vi "RadioFM.vi"() -> ()   [LabVIEW 2019]
uses:
  <vilib>/Analysis/3filter.llb/Filter Passband Type.ctl
  <vilib>/Waveform/WDTOps.llb/WDT Get Waveform Time Array DBL.vi
  <vilib>/Analysis/3filter.llb/Butterworth Filter (DBL).vi
  <vilib>/measure/maspectr.llb/FFT Power Spectrum and PSD for 1 Chan.vi
  <vilib>/Waveform/WDTOps.llb/WDT Waveform Duration DBL.vi
  <vilib>/Waveform/WDTOps.llb/WDT Get Waveform Subset DBL.vi
  <vilib>/measure/NI_MABase.lvlib
  <vilib>/measure/NI_MAPro.lvlib
  <vilib>/Analysis/NI_AALBase.lvlib
  <vilib>/Analysis/NI_AALPro.lvlib
panel:
  out "Sampling Info":cluster{dbl, dbl}={705600.0, 1411200.0}
  out "dt":dbl=1.417233560090703e-06
  in  "Tab Control 2":T1(tab)
  out "Espectro del Canal":cluster{"f0":dbl, "df":dbl, "magnitude":dbl[]}(graph)={"f0"=0.0, "df"=0.5, "magnitude"=[]}
  out "Espectro Recibido":cluster{"f0":dbl, "df":dbl, "magnitude":dbl[]}(graph)={"f0"=0.0, "df"=0.5, "magnitude"=[]}
  out "Señal Recibida":waveform(dbl)(graph)={"t0"=timestamp(0 s since 1904-01-01), "dt"=1.417233560090703e-06, "Y"=[]}
  out "Espectro Mezclador":cluster{"f0":dbl, "df":dbl, "magnitude":dbl[]}(graph)={"f0"=0.0, "df"=0.5, "magnitude"=[]}
  out "Espectro Detectado":cluster{"f0":dbl, "df":dbl, "magnitude":dbl[]}(graph)={"f0"=0.0, "df"=0.5, "magnitude"=[]}
  out "Señal Detectada":waveform(dbl)(graph)={"t0"=timestamp(0 s since 1904-01-01), "dt"=1.417233560090703e-06, "Y"=[]}
  out "Señal Recuperada":waveform(dbl)(graph)={"t0"=timestamp(0.4 s since 1904-01-01), "dt"=1.417233560090703e-06, "Y"=[]}
  out "Espectro Recuperado":cluster{"f0":dbl, "df":dbl, "magnitude":dbl[]}(graph)={"f0"=0.0, "df"=0.6250005536073497, "magnitude"=[]}
  in  "Sintonizador":cluster{"Emisora":dbl, "Volumen":dbl}={"Emisora"=65050.0, "Volumen"=5.081596097153018} {"Volumen" scale=0.0..10.0; "Emisora" scale=44050.0..65050.0}
  in  "stop":bool
  in  "Tab Control":enum32{"Page 1", "Page 2", "Page 3", "Page 4"}(tab)
  out "Beta":dbl=0.003302742812078559
  out "Espectro Emisora":cluster{"f0":dbl, "df":dbl, "magnitude":dbl[]}(graph)={"f0"=0.0, "df"=0.5, "magnitude"=[]}
  in  "Mensaje 1":T2={"Fase"=0.0, "Frecuencia"=1513.8932349543995, "Amplitud"=5.617529880478088, "Kf"=5.0} {"Amplitud" scale=0.0..100.0; "Frecuencia" scale=1.0..5000.0; "Fase" scale=0.0..90.0}
  out "Emisora 1":waveform(dbl)(graph)={"t0"=timestamp(232 s since 1904-01-01), "dt"=1.417233560090703e-06, "Y"=[]}
  out "Beta 2":dbl=16.18677363495819
  out "Emisora 2":waveform(dbl)(graph)={"t0"=timestamp(232 s since 1904-01-01), "dt"=1.417233560090703e-06, "Y"=[]}
  in  "Mensaje 2":T2={"Fase"=0.0, "Frecuencia"=308.8941695707426, "Amplitud"=5.0199203187251, "Kf"=5000.0} {"Amplitud" scale=0.0..100.0; "Frecuencia" scale=0.0..1000.0; "Fase" scale=0.0..10.0}
  out "Espectro Emisora 2":cluster{"f0":dbl, "df":dbl, "magnitude":dbl[]}(graph)={"f0"=0.0, "df"=0.5, "magnitude"=[]}
  out "Beta 3":dbl=14.81360563253253
  out "Emisora 3":waveform(dbl)(graph)={"t0"=timestamp(232 s since 1904-01-01), "dt"=1.417233560090703e-06, "Y"=[]}
  in  "Mensaje 3":T2={"Fase"=0.0, "Frecuencia"=337.5275489324068, "Amplitud"=5.0199203187251, "Kf"=5000.0} {"Amplitud" scale=0.0..100.0; "Frecuencia" scale=0.0..1000.0; "Fase" scale=0.0..10.0}
  out "Espectro Emisora 3":cluster{"f0":dbl, "df":dbl, "magnitude":dbl[]}(graph)={"f0"=0.0, "df"=0.5, "magnitude"=[]}
  out "Beta 4":dbl=0.058823529411764705
  out "Emisora 4":waveform(dbl)(graph)={"t0"=timestamp(0 s since 1904-01-01), "dt"=1.417233560090703e-06, "Y"=[]}
  in  "Mensaje 4":cluster{"Amplitud":dbl, "Kf":dbl}={"Amplitud"=5.016722408026756, "Kf"=200.0} {"Amplitud" scale=0.0..100.0}
  out "Espectro Emisora 4":cluster{"f0":dbl, "df":dbl, "magnitude":dbl[]}(graph)={"f0"=0.0, "df"=0.4778519417475728, "magnitude"=[]}
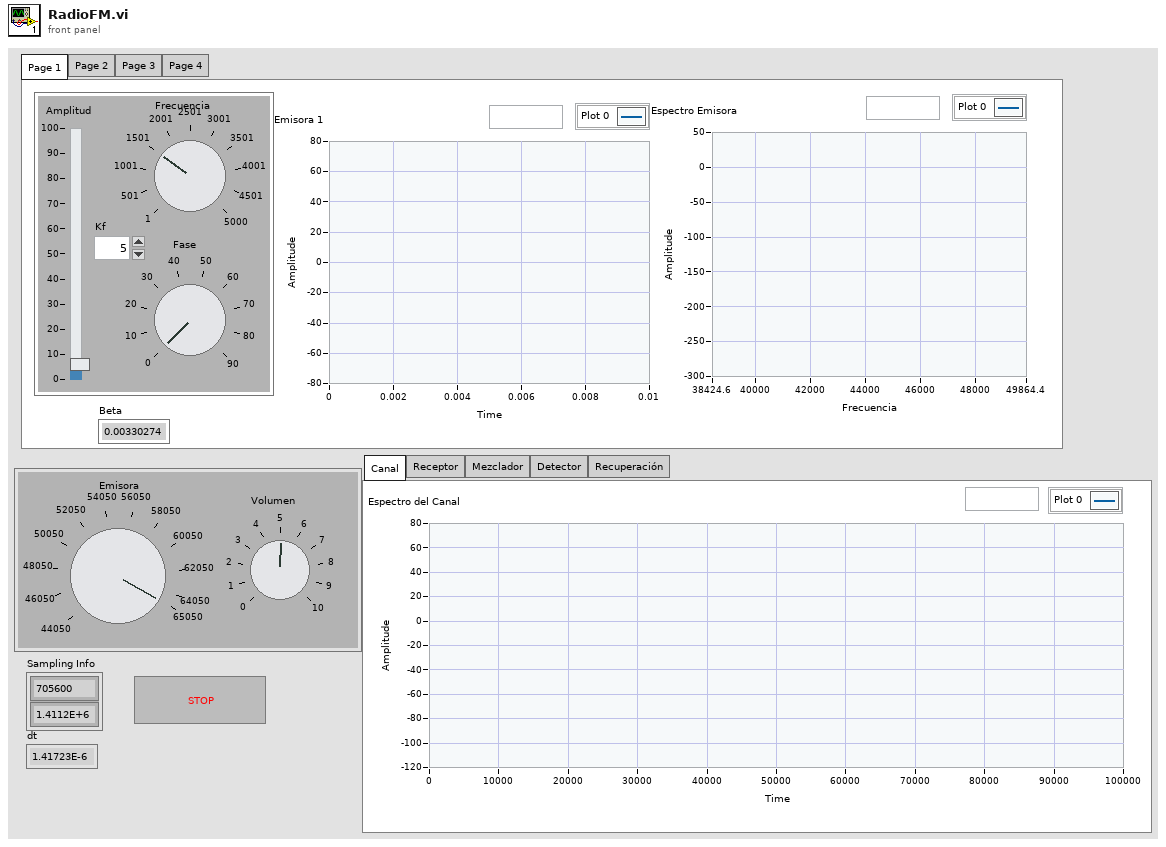
[diagram p1: front panel]
types:
  T1 = enum32{"Canal", "Receptor", "Mezclador", "Detector", "Recuperación"}
  T2 = cluster{"Fase":dbl, "Frecuencia":dbl, "Amplitud":dbl, "Kf":dbl}
  T3 = typedef "NI_AALBase.lvlib/Filter Passband Type.ctl" = enum32{"Lowpass", "Highpass", "Bandpass", "Bandstop"}
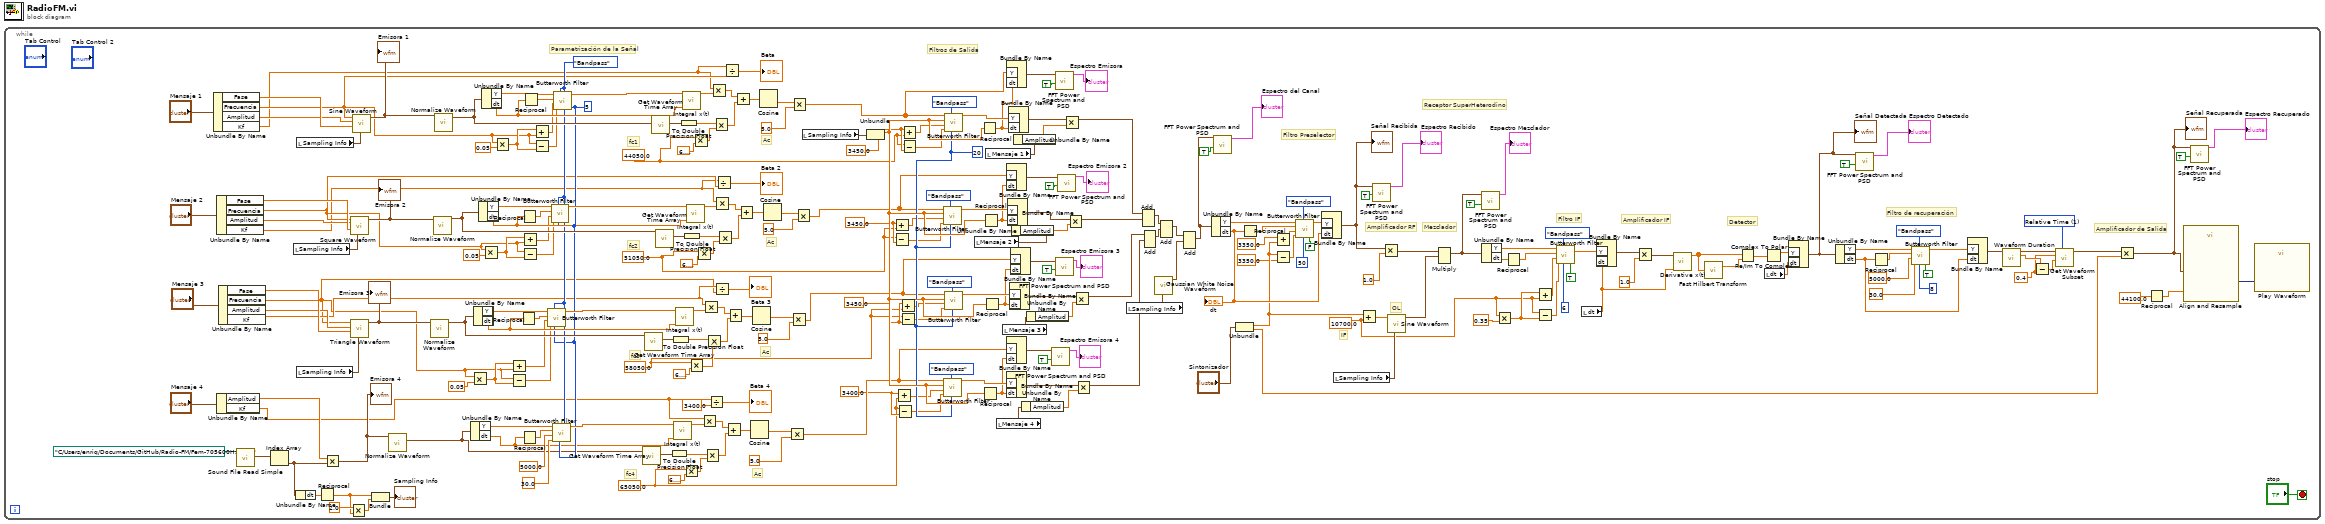
[diagram p0: block diagram]
diagram:
  n1 = while {
    stop <- "stop" stop-if-true
    w15 = 44050.0 ("y")
    w20 = 3450.0 ("x")
    w16 = 51050.0 ("x")
    w23 = 3450.0 ("x+y")
    w17 = 58050.0 ("y")
    w27 = 3450.0 ("y")
    w26 = 3400.0 ("y")
    w18 = 65050.0
    w43 = u16 1 items=["Samples", "Relative Time"] ("start/duration format")
    w49 = 0.4 ("start samples/time")
    w102 = 5 ("order")
    w107 = Filter_Passband_Type."Bandpass" ("filter type")
    w160 = 20 ("order")
    w80 = 10700.0 ("y")
    # "Amplificador de Salida"
    # "Parametrización de la Señal"
    # "Filtro IF"
    # "Filtro de recuperación"
    # "Amplificador RF"
    # "Amplificador IF"
    # "Detector"
    # "Mezclador"
    # "Receptor SuperHeterodino"
    # "Filtros de Salida"
    # "Ac"
    # "fc4"
    # "Ac"
    # "fc3"
    # "Ac"
    # "fc2"
    # "Ac"
    # "fc1"
    # "Filtro Preselector"
    # "IF"
    # "OL"
    n2 = Unbundle By Name("Mensaje 1") -> ("Fase"=w218:dbl, "Frecuencia"=w63:dbl, "Amplitud"=w210:dbl, "Kf"=w62:dbl)
    n3 = Unbundle By Name("Mensaje 2") -> ("Fase"=w216:dbl, "Frecuencia"=w61:dbl, "Amplitud"=w197:dbl, "Kf"=w60:dbl)
    n4 = Unbundle By Name("Mensaje 4") -> ("Amplitud"=w211:dbl, "Kf"=w57:dbl)
    n5 = Unbundle By Name("Mensaje 3") -> ("Fase"=w214:dbl, "Frecuencia"=w58:dbl, "Amplitud"=w171:dbl, "Kf"=w59:dbl)
    n6 = call <vilib>:"Sound File Read Simple.vi"("path"=path "C:/Users/enriq/Documents/GitHub/Radio-FM/Fem-705600Hz.wav") -> ("data"=w257:waveform(dbl)[])  [unwired: 7 in, 3 out]
    n7 = Index Array(array=w257) -> (element=w212:waveform(dbl))  [unwired: 1 in]
    n8 = local read "Sampling Info"() -> (w241:cluster{dbl, dbl})
    n9 = Unbundle By Name(w212) -> ("dt"=w256:dbl)
    n10 = local read "Sampling Info"() -> (w242:cluster{dbl, dbl})
    n11 = local read "Sampling Info"() -> (w253:cluster{dbl, dbl})
    n12 = Reciprocal(x=w256) -> (1/x=w170:dbl)
    n13 = Multiply(x=w211, y=w212) -> (x*y=w72:waveform(dbl))
    "Emisora 4" <- w72
    n14 = Multiply(x=2.0, y=w170) -> (x*y=w254:dbl)
    n15 = call <vilib>:"Square Waveform.vi"("sampling info"=w241, "phase"=w216, "amplitude"=w197, "frequency"=w61) -> ("signal out"=w196:waveform(dbl))  [unwired: 6 in, 1 out]
    "Emisora 2" <- w196
    n16 = call <vilib>:"Triangle Waveform.vi"("sampling info"=w242, "phase"=w214, "amplitude"=w171, "frequency"=w58) -> ("signal out"=w172:waveform(dbl))  [unwired: 6 in, 1 out]
    "Emisora 3" <- w172
    n17 = call <vilib>:"Sine Waveform.vi"("sampling info"=w253, "phase"=w218, "amplitude"=w210, "frequency"=w63) -> ("signal out"=w139:waveform(dbl))  [unwired: 6 in, 1 out]
    "Emisora 1" <- w139
    n18 = Bundle(w170, w254) -> (→"Sampling Info":cluster{dbl, dbl})  [unwired: 1 in]
    n19 = call <vilib>:"Normalize Waveform.vi"("waveform in"=w72) -> ("normalized waveform"=w44:waveform(dbl))  [unwired: 7 in, 3 out]
    n20 = call <vilib>:"Normalize Waveform.vi"("waveform in"=w172) -> ("normalized waveform"=w136:waveform(dbl))  [unwired: 7 in, 3 out]
    n21 = call <vilib>:"Normalize Waveform.vi"("waveform in"=w196) -> ("normalized waveform"=w137:waveform(dbl))  [unwired: 7 in, 3 out]
    n22 = call <vilib>:"Normalize Waveform.vi"("waveform in"=w139) -> ("normalized waveform"=w138:waveform(dbl))  [unwired: 7 in, 3 out]
    n23 = Unbundle By Name(w44) -> ("Y"=w173:dbl[], "dt"=w78:dbl)
    n24 = Multiply(x=w58, y=0.05) -> (x*y=w123:dbl)
    n25 = Unbundle By Name(w136) -> ("Y"=w194:dbl[], "dt"=w115:dbl)
    n26 = Unbundle By Name(w137) -> ("Y"=w198:dbl[], "dt"=w114:dbl)
    n27 = Unbundle By Name(w138) -> ("Y"=w226:dbl[], "dt"=w130:dbl)
    n28 = Multiply(x=w61, y=0.05) -> (x*y=w124:dbl)
    n29 = Multiply(x=w63, y=0.05) -> (x*y=w129:dbl)
    n30 = Add(x=w123, y=w58) -> (x+y=w109:dbl)
    n31 = Subtract(x=w58, y=w123) -> (x-y=w108:dbl)
    n32 = Reciprocal(x=w115) -> (1/x=w117:dbl)
    n33 = Reciprocal(x=w114) -> (1/x=w118:dbl)
    n34 = Reciprocal(x=w78) -> (1/x=w116:dbl)
    n35 = Add(x=w124, y=w61) -> (x+y=w113:dbl)
    n36 = Subtract(x=w61, y=w124) -> (x-y=w112:dbl)
    n37 = Reciprocal(x=w130) -> (1/x=w131:dbl)
    n38 = Add(x=w129, y=w63) -> (x+y=w127:dbl)
    n39 = Subtract(x=w63, y=w129) -> (x-y=w126:dbl)
    n40 = call-poly <vilib>:"Butterworth Filter.vi"("order"=w102, "filter type"=w107, "low cutoff freq: fl"=w108, "high cutoff freq: fh"=w109, "sampling freq: fs"=w117, "X"=w194) -> ("Filtered X"=w120:dbl[])  [unwired: 2 in, 1 out]
    n41 = call-poly <vilib>:"Butterworth Filter.vi"("order"=w102, "filter type"=w107, "low cutoff freq: fl"=w112, "high cutoff freq: fh"=w113, "sampling freq: fs"=w118, "X"=w198) -> ("Filtered X"=w121:dbl[])  [unwired: 2 in, 1 out]
    n42 = call-poly <vilib>:"Butterworth Filter.vi"("order"=w102, "filter type"=w107, "low cutoff freq: fl"=30.0, "high cutoff freq: fh"=5000.0, "sampling freq: fs"=w116, "X"=w173) -> ("Filtered X"=w119:dbl[])  [unwired: 2 in, 1 out]
    n43 = call-poly <vilib>:"Butterworth Filter.vi"("order"=w102, "filter type"=w107, "low cutoff freq: fl"=w126, "high cutoff freq: fh"=w127, "sampling freq: fs"=w131, "X"=w226) -> ("Filtered X"=w132:dbl[])  [unwired: 2 in, 1 out]
    n44 = call-poly <vilib>:"Get Waveform Time Array.vi"("waveform in"=w44) -> ("X array"=w178:timestamp[])  [unwired: 9 in, 1 out]
    n45 = call-poly <vilib>:"Get Waveform Time Array.vi"("waveform in"=w136) -> ("X array"=w189:timestamp[])  [unwired: 9 in, 1 out]
    n46 = call-poly <vilib>:"Get Waveform Time Array.vi"("waveform in"=w138) -> ("X array"=w227:timestamp[])  [unwired: 9 in, 1 out]
    n47 = call-poly <vilib>:"Get Waveform Time Array.vi"("waveform in"=w137) -> ("X array"=w203:timestamp[])  [unwired: 9 in, 1 out]
    n48 = To Double Precision Float(number=w178) -> (double precision float=w177:dbl[])
    n49 = To Double Precision Float(number=w189) -> (double precision float=w190:dbl[])
    n50 = call <vilib>:"Integral x(t).vi"("dt"=w78, "X"=w119) -> ("Integral X"=w179:dbl[])  [unwired: 8 in, 1 out]
    n51 = call <vilib>:"Integral x(t).vi"("dt"=w115, "X"=w120) -> ("Integral X"=w188:dbl[])  [unwired: 8 in, 1 out]
    n52 = To Double Precision Float(number=w227) -> (double precision float=w228:dbl[])
    n53 = call <vilib>:"Integral x(t).vi"("dt"=w130, "X"=w132) -> ("Integral X"=w225:dbl[])  [unwired: 8 in, 1 out]
    n54 = Multiply(x=w18, y=6.283185307179586) -> (x*y=w174:dbl)
    n55 = To Double Precision Float(number=w203) -> (double precision float=w202:dbl[])
    n56 = call <vilib>:"Integral x(t).vi"("dt"=w114, "X"=w121) -> ("Integral X"=w204:dbl[])  [unwired: 8 in, 1 out]
    n57 = Multiply(x=w17, y=6.283185307179586) -> (x*y=w193:dbl)
    n58 = Multiply(x=w15, y=6.283185307179586) -> (x*y=w230:dbl)
    n59 = Multiply(x=w16, y=6.283185307179586) -> (x*y=w199:dbl)
    n60 = Multiply(x=w57, y=w179) -> (x*y=w176:dbl[])
    n61 = Multiply(x=w59, y=w188) -> (x*y=w191:dbl[])
    n62 = Multiply(x=w177, y=w174) -> (x*y=w175:dbl[])
    n63 = Multiply(x=w190, y=w193) -> (x*y=w192:dbl[])
    n64 = Divide(x=w57, y=3400.0) -> (x/y=→"Beta 4":dbl)
    n65 = Multiply(x=w62, y=w225) -> (x*y=w64:dbl[])
    n66 = Multiply(x=w228, y=w230) -> (x*y=w229:dbl[])
    n67 = Multiply(x=w60, y=w204) -> (x*y=w201:dbl[])
    n68 = Divide(x=w59, y=w58) -> (x/y=→"Beta 3":dbl)
    n69 = Divide(x=w60, y=w61) -> (x/y=→"Beta 2":dbl)
    n70 = Multiply(x=w202, y=w199) -> (x*y=w200:dbl[])
    n71 = Divide(x=w62, y=w63) -> (x/y=→"Beta":dbl)
    n72 = Add(x=w176, y=w175) -> (x+y=w180:dbl[])
    n73 = Add(x=w191, y=w192) -> (x+y=w187:dbl[])
    n74 = Add(x=w64, y=w229) -> (x+y=w224:dbl[])
    n75 = Add(x=w201, y=w200) -> (x+y=w205:dbl[])
    n76 = Cosine(x=w180) -> (cos(x)=w181:dbl[])
    n77 = Cosine(x=w187) -> (cos(x)=w186:dbl[])
    n78 = Cosine(x=w224) -> (cos(x)=w223:dbl[])
    n79 = Cosine(x=w205) -> (cos(x)=w206:dbl[])
    n80 = Multiply(x=w181, y=5.0) -> (x*y=w87:dbl[])
    n81 = Multiply(x=w186, y=5.0) -> (x*y=w88:dbl[])
    n82 = Multiply(x=w223, y=5.0) -> (x*y=w142:dbl[])
    n83 = Multiply(x=w206, y=5.0) -> (x*y=w92:dbl[])
    n84 = local read "Sampling Info"() -> (w164:cluster{dbl, dbl})
    n85 = Unbundle(w164) -> (w195:dbl)  [unwired: 1 out]
    n86 = Add(x=w23, y=w16) -> (x+y=w25:dbl)
    n87 = Subtract(x=w16, y=w23) -> (x-y=w24:dbl)
    n88 = Add(x=w26, y=w18) -> (x+y=w31:dbl)
    n89 = Subtract(x=w18, y=w26) -> (x-y=w30:dbl)
    n90 = Add(x=w27, y=w17) -> (x+y=w29:dbl)
    n91 = Subtract(x=w17, y=w27) -> (x-y=w28:dbl)
    n92 = Add(x=w20, y=w15) -> (x+y=w22:dbl)
    n93 = Subtract(x=w15, y=w20) -> (x-y=w21:dbl)
    n94 = call-poly <vilib>:"Butterworth Filter.vi"("order"=w160, "filter type"=Filter_Passband_Type."Bandpass", "low cutoff freq: fl"=w24, "high cutoff freq: fh"=w25, "sampling freq: fs"=w195, "X"=w92) -> ("Filtered X"=w168:dbl[])  [unwired: 2 in, 1 out]
    n95 = call-poly <vilib>:"Butterworth Filter.vi"("order"=w160, "filter type"=Filter_Passband_Type."Bandpass", "low cutoff freq: fl"=w30, "high cutoff freq: fh"=w31, "sampling freq: fs"=w195, "X"=w87) -> ("Filtered X"=w166:dbl[])  [unwired: 2 in, 1 out]
    n96 = call-poly <vilib>:"Butterworth Filter.vi"("order"=w160, "filter type"=Filter_Passband_Type."Bandpass", "low cutoff freq: fl"=w21, "high cutoff freq: fh"=w22, "sampling freq: fs"=w195, "X"=w142) -> ("Filtered X"=w169:dbl[])  [unwired: 2 in, 1 out]
    n97 = call-poly <vilib>:"Butterworth Filter.vi"("order"=w160, "filter type"=Filter_Passband_Type."Bandpass", "low cutoff freq: fl"=w28, "high cutoff freq: fh"=w29, "sampling freq: fs"=w195, "X"=w88) -> ("Filtered X"=w167:dbl[])  [unwired: 2 in, 1 out]
    n98 = local read "Mensaje 2"() -> (w4:T2)
    n99 = Reciprocal(x=w195) -> (1/x=w141:dbl)
    n100 = Reciprocal(x=w195) -> (1/x=w86:dbl)
    n101 = Reciprocal(x=w195) -> (1/x=w91:dbl)
    n102 = Reciprocal(x=w195) -> (1/x=w89:dbl)
    n103 = local read "Mensaje 1"() -> (w2:T2)
    n104 = local read "Mensaje 4"() -> (w8:cluster{"Amplitud":dbl, "Kf":dbl})
    n105 = local read "Mensaje 3"() -> (w6:T2)
    n106 = Bundle By Name("Y"=w92, "dt"=w91) -> (w93:waveform(dbl))  [unwired: 1 in]
    n107 = Bundle By Name("Y"=w87, "dt"=w86) -> (w40:waveform(dbl))  [unwired: 1 in]
    n108 = Bundle By Name("Y"=w166, "dt"=w86) -> (w19:waveform(dbl))  [unwired: 1 in]
    n109 = Bundle By Name("Y"=w142, "dt"=w141) -> (w48:waveform(dbl))  [unwired: 1 in]
    n110 = Bundle By Name("Y"=w168, "dt"=w91) -> (w143:waveform(dbl))  [unwired: 1 in]
    n111 = Bundle By Name("Y"=w169, "dt"=w141) -> (w47:waveform(dbl))  [unwired: 1 in]
    n112 = Bundle By Name("Y"=w167, "dt"=w89) -> (w243:waveform(dbl))  [unwired: 1 in]
    n113 = Bundle By Name("Y"=w88, "dt"=w89) -> (w90:waveform(dbl))  [unwired: 1 in]
    n114 = Unbundle By Name(w4) -> ("Amplitud"=w3:dbl)
    n115 = Unbundle By Name(w2) -> ("Amplitud"=w1:dbl)
    n116 = Unbundle By Name(w8) -> ("Amplitud"=w7:dbl)
    n117 = Unbundle By Name(w6) -> ("Amplitud"=w5:dbl)
    n118 = call-poly <vilib>:"FFT Power Spectrum and PSD.vi"("dB On (F)"=TRUE, "time signal"=w40) -> ("Power Spectrum / PSD"=→"Espectro Emisora 4":cluster{"f0":dbl, "df":dbl, "magnitude":dbl[]})  [unwired: 6 in, 3 out]
    n119 = call-poly <vilib>:"FFT Power Spectrum and PSD.vi"("dB On (F)"=TRUE, "time signal"=w48) -> ("Power Spectrum / PSD"=→"Espectro Emisora":cluster{"f0":dbl, "df":dbl, "magnitude":dbl[]})  [unwired: 6 in, 3 out]
    n120 = call-poly <vilib>:"FFT Power Spectrum and PSD.vi"("dB On (F)"=TRUE, "time signal"=w90) -> ("Power Spectrum / PSD"=→"Espectro Emisora 3":cluster{"f0":dbl, "df":dbl, "magnitude":dbl[]})  [unwired: 6 in, 3 out]
    n121 = call-poly <vilib>:"FFT Power Spectrum and PSD.vi"("dB On (F)"=TRUE, "time signal"=w93) -> ("Power Spectrum / PSD"=→"Espectro Emisora 2":cluster{"f0":dbl, "df":dbl, "magnitude":dbl[]})  [unwired: 6 in, 3 out]
    n122 = Multiply(x=w47, y=w1) -> (x*y=w12:waveform(dbl))
    n123 = Multiply(x=w143, y=w3) -> (x*y=w11:waveform(dbl))
    n124 = Multiply(x=w243, y=w5) -> (x*y=w10:waveform(dbl))
    n125 = Multiply(x=w19, y=w7) -> (x*y=w9:waveform(dbl))
    n126 = local read "Sampling Info"() -> (w103:cluster{dbl, dbl})
    n127 = Add(1:w11, 2:w12) -> (0:w245:waveform(dbl))  [unwired: 1 in, 1 out]
    n128 = Add(1:w9, 2:w10) -> (0:w244:waveform(dbl))  [unwired: 1 in, 1 out]
    n129 = call <vilib>:"Gaussian White Noise Waveform.vi"("sampling info"=w103) -> ("signal out"=w104:waveform(dbl))  [unwired: 9 in, 1 out]
    n130 = Add(1:w244, 2:w245) -> (0:w14:waveform(dbl))  [unwired: 1 in, 1 out]
    n131 = Add(1:w104, 2:w14) -> (0:w13:waveform(dbl))  [unwired: 1 in, 1 out]
    n132 = Unbundle By Name(w13) -> ("Y"=w237:dbl[], "dt"=w140:dbl)
    "dt" <- w140
    n133 = call-poly <vilib>:"FFT Power Spectrum and PSD.vi"("dB On (F)"=TRUE, "time signal"=w13) -> ("Power Spectrum / PSD"=→"Espectro del Canal":cluster{"f0":dbl, "df":dbl, "magnitude":dbl[]})  [unwired: 6 in, 3 out]
    n134 = Unbundle("Sintonizador") -> ("Emisora"=w133:dbl, "Volumen"=w105:dbl)
    n135 = Reciprocal(x=w140) -> (1/x=w236:dbl)
    n136 = Add(x=3350.0, y=w133) -> (x+y=w235:dbl)
    n137 = Subtract(x=w133, y=3350.0) -> (x-y=w165:dbl)
    n138 = call-poly <vilib>:"Butterworth Filter.vi"("init/cont (init:F)"=FALSE, "order"=50, "filter type"=Filter_Passband_Type."Bandpass", "low cutoff freq: fl"=w165, "high cutoff freq: fh"=w235, "sampling freq: fs"=w236, "X"=w237) -> ("Filtered X"=w238:dbl[])  [unwired: 1 in, 1 out]
    n139 = Bundle By Name("Y"=w238, "dt"=w140) -> (w70:waveform(dbl))  [unwired: 1 in]
    "Señal Recibida" <- w70
    n140 = local read "Sampling Info"() -> (w159:cluster{dbl, dbl})
    n141 = Add(x=w133, y=w80) -> (x+y=w234:dbl)
    n142 = call-poly <vilib>:"FFT Power Spectrum and PSD.vi"("dB On (F)"=TRUE, "time signal"=w70) -> ("Power Spectrum / PSD"=→"Espectro Recibido":cluster{"f0":dbl, "df":dbl, "magnitude":dbl[]})  [unwired: 6 in, 3 out]
    n143 = Multiply(x=w70, y=1.0) -> (x*y=w233:waveform(dbl))
    n144 = call <vilib>:"Sine Waveform.vi"("sampling info"=w159, "frequency"=w234) -> ("signal out"=w38:waveform(dbl))  [unwired: 8 in, 1 out]
    n145 = Multiply(1:w38, 2:w233) -> (0:w71:waveform(dbl))  [unwired: 1 in, 1 out]
    n146 = call-poly <vilib>:"FFT Power Spectrum and PSD.vi"("dB On (F)"=TRUE, "time signal"=w71) -> ("Power Spectrum / PSD"=→"Espectro Mezclador":cluster{"f0":dbl, "df":dbl, "magnitude":dbl[]})  [unwired: 6 in, 3 out]
    n147 = Unbundle By Name(w71) -> ("Y"=w154:dbl[], "dt"=w155:dbl)
    n148 = Multiply(x=w80, y=0.35) -> (x*y=w134:dbl)
    n149 = Reciprocal(x=w155) -> (1/x=w153:dbl)
    n150 = Add(x=w134, y=w80) -> (x+y=w152:dbl)
    n151 = Subtract(x=w80, y=w134) -> (x-y=w151:dbl)
    n152 = call-poly <vilib>:"Butterworth Filter.vi"("init/cont (init:F)"=TRUE, "order"=6, "filter type"=Filter_Passband_Type."Bandpass", "low cutoff freq: fl"=w151, "high cutoff freq: fh"=w152, "sampling freq: fs"=w153, "X"=w154) -> ("Filtered X"=w146:dbl[])  [unwired: 1 in, 1 out]
    n153 = local read "dt"() -> (w73:dbl)
    n154 = Bundle By Name("Y"=w146, "dt"=w73) -> (w69:waveform(dbl))  [unwired: 1 in]
    n155 = Multiply(x=w69, y=1.0) -> (x*y=w81:waveform(dbl))
    n156 = call <vilib>:"Derivative x(t).vi"("dt"=w73, "X"=w81) -> ("dX/dt"=w74:dbl[])  [unwired: 8 in, 1 out]
    n157 = call <vilib>:"Fast Hilbert Transform.vi"("X"=w74) -> ("Hilbert{X}"=w76:dbl[])  [unwired: 1 out]
    n158 = Re/Im To Complex(1:w76, 2:w74) -> (0:w77:cdb[])
    n159 = local read "dt"() -> (w145:dbl)
    n160 = Complex To Polar(r * e^(i*theta)=w77) -> (r=w75:dbl[])  [unwired: 1 out]
    n161 = Bundle By Name("Y"=w75, "dt"=w145) -> (w65:waveform(dbl))  [unwired: 1 in]
    "Señal Detectada" <- w65
    n162 = Unbundle By Name(w65) -> ("Y"=w147:dbl[], "dt"=w79:dbl)
    n163 = call-poly <vilib>:"FFT Power Spectrum and PSD.vi"("dB On (F)"=TRUE, "time signal"=w65) -> ("Power Spectrum / PSD"=→"Espectro Detectado":cluster{"f0":dbl, "df":dbl, "magnitude":dbl[]})  [unwired: 6 in, 3 out]
    n164 = Reciprocal(x=w79) -> (1/x=w158:dbl)
    n165 = call-poly <vilib>:"Butterworth Filter.vi"("init/cont (init:F)"=TRUE, "order"=8, "filter type"=Filter_Passband_Type."Bandpass", "low cutoff freq: fl"=30.0, "high cutoff freq: fh"=5000.0, "sampling freq: fs"=w158, "X"=w147) -> ("Filtered X"=w144:dbl[])  [unwired: 1 in, 1 out]
    n166 = Bundle By Name("Y"=w144, "dt"=w79) -> (w35:waveform(dbl))  [unwired: 1 in]
    n167 = call-poly <vilib>:"Waveform Duration.vi"("waveform in"=w35) -> ("duration"=w51:dbl, "waveform out"=w39:waveform(dbl))  [unwired: 8 in, 1 out]
    n168 = Subtract(x=w51, y=w49) -> (x-y=w50:dbl)
    n169 = call-poly <vilib>:"Get Waveform Subset.vi"("start/duration format"=w43, "duration"=w50, "start samples/time"=w49, "waveform in"=w39) -> ("waveform out"=w34:waveform(dbl))  [unwired: 2 in, 3 out]
    n170 = Multiply(x=w34, y=w105) -> (x*y=w41:waveform(dbl))
    "Señal Recuperada" <- w41
    n171 = Reciprocal(x=44100.0 ("dt")) -> (1/x=w46:dbl)
    n172 = call "Align and Resample"("dt"=w46, "Signals"=w41) -> ("Resampled Signals"=w42:dynamicdata)  [unwired: 7 in, 2 out]
    n173 = call-poly <vilib>:"FFT Power Spectrum and PSD.vi"("dB On (F)"=TRUE, "time signal"=w41) -> ("Power Spectrum / PSD"=→"Espectro Recuperado":cluster{"f0":dbl, "df":dbl, "magnitude":dbl[]})  [unwired: 6 in, 3 out]
    n174 = call "Play Waveform"("Data"=w42) -> ()  [unwired: 18 in, 1 out]
  }
